vi "数字键盘.vi"(8 "错误输入":errorcluster caption="错误输入（无错误）", 11 "数值输入":string) -> (0 "错误输出":errorcluster, 3 "数值输出":string)   [LabVIEW 2014]
panel:
  in  "数字按钮":T1
  in  "放弃按钮":bool
  in  "删除":bool
  in  "清空":bool
  in  "确定按钮":bool
  in  "负号":bool
  in  "0":bool
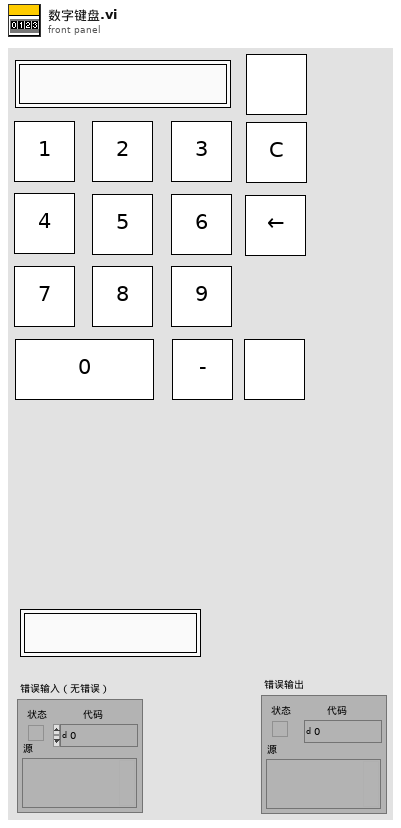
[diagram p1: front panel]
types:
  T1 = cluster{"1":bool, "2":bool, "3":bool, "4":bool, "5":bool, "6":bool, "7":bool, "8":bool, "9":bool}
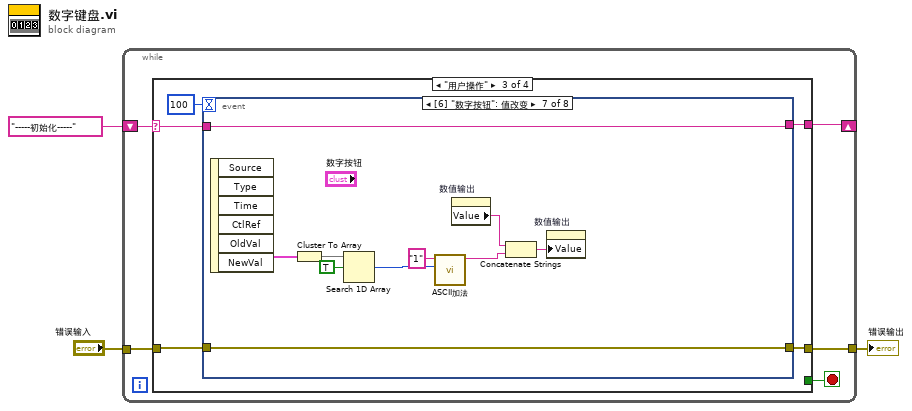
[diagram p0: block diagram]
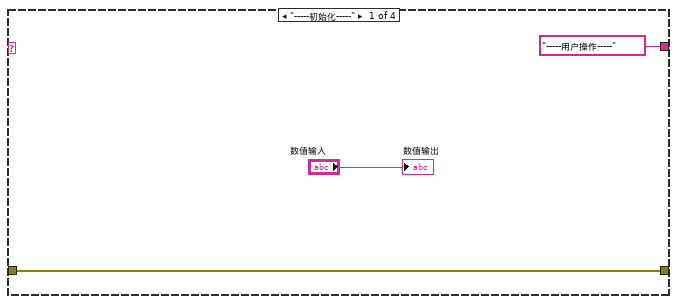
[diagram p2: hidden frame]
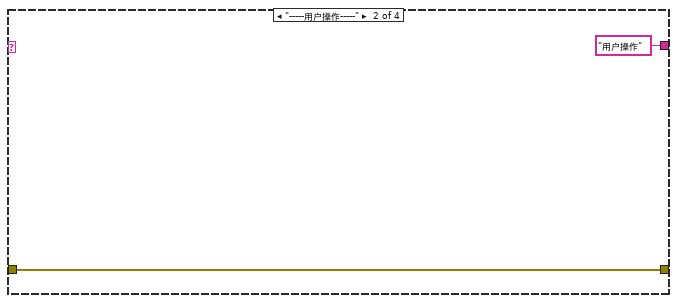
[diagram p3: hidden frame]
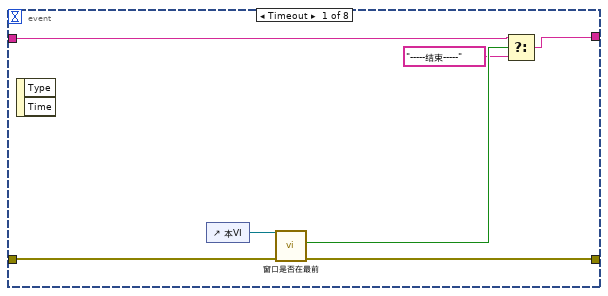
[diagram p4: hidden frame]
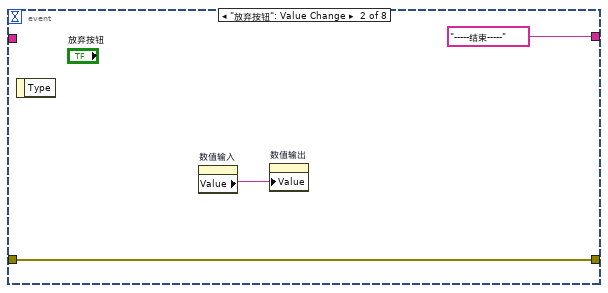
[diagram p5: hidden frame]
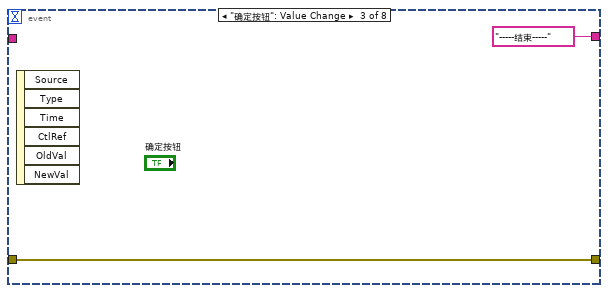
[diagram p6: hidden frame]
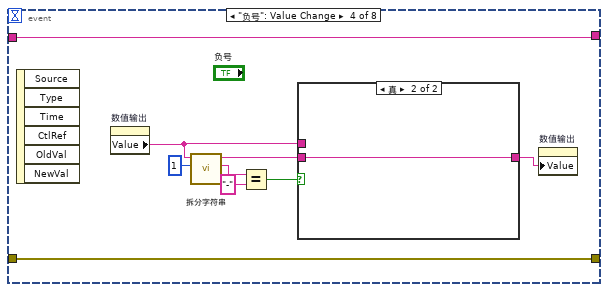
[diagram p7: hidden frame]
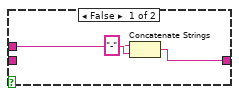
[diagram p8: hidden frame]
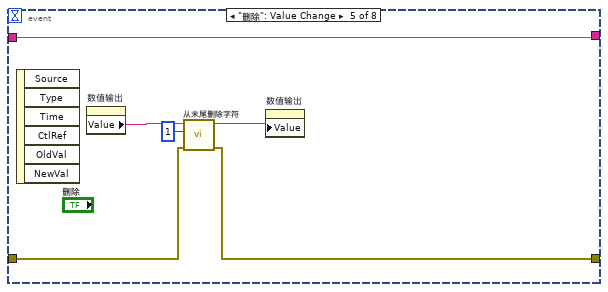
[diagram p9: hidden frame]
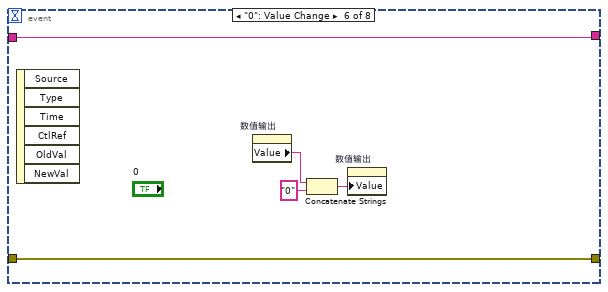
[diagram p10: hidden frame]
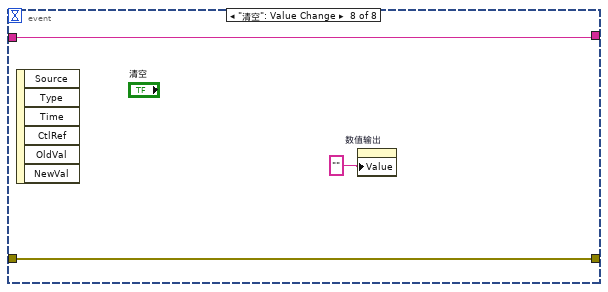
[diagram p11: hidden frame]
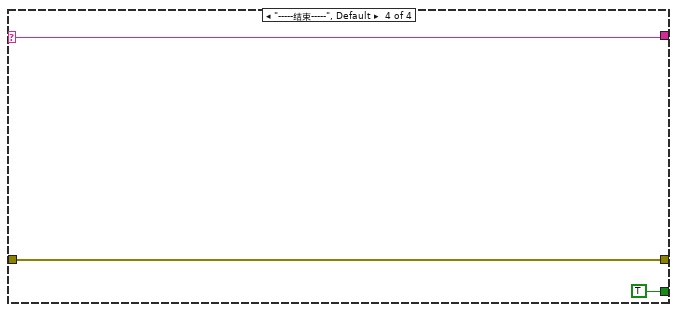
[diagram p12: hidden frame]
diagram:
  n1 = while {
    tunnel: [w8] -> w2
    tunnel: "错误输入" -> [w7]
    shift-right: [w4] -> _
    shift-left: "-----初始化-----" -> [w6]
    stop <- w5 stop-if-true
    n2 = case shown="\"用户操作\"" w6 {
      selector: w6 -> [_ _ w15 w68]
      tunnel: [w11 w12 w18 w70] -> w8
      tunnel: w7 -> [w11 w12 w17 w70]
      tunnel: [_ _ _ TRUE] -> w5
      tunnel: ["-----用户操作-----" "用户操作" w16 w68] -> w4
      frame "-----初始化-----" {
        "数值输出" <- "数值输入"
      }
      frame "-----用户操作-----" {
      }
      frame "用户操作" {
        n3 = event shown="[6] \"数字按钮\": 值改变" {
          selector: _ -> [_ _ _ _ _ _ _ _]
          dyn-events: _ -> [_ _ _ _ _ _ _ _]
          timeout: 100 -> [_ _ _ _ _ _ _ _]
          tunnel: [w24 w27 w30 w38 w45 w53 w64 w66] -> w18
          tunnel: w17 -> [w25 w27 w30 w38 w46 w53 w64 w66]
          tunnel: [w21 "-----结束-----" "-----结束-----" w39 w49 w54 w63 w67] -> w16
          tunnel: w15 -> [w22 _ _ w39 w49 w54 w63 w67]
          event Timeout {
            n4 = event-data() -> ()  [unwired: 1 in, 2 out]
            n5 = control-ref of="本VI"() -> (w19:refnum<vi>)
            n6 = call "窗口是否在最前.vi"("错误输入（无错误）"=w25, "引用"=w19) -> ("错误输出"=w24:errorcluster, "在最前？"=w23:bool)  [unwired: 7 in, 1 out]
            n7 = Select(t=w22, s=w23, f="-----结束-----") -> (s? t:f=w21:string)
          }
          event "放弃按钮": Value Change {
            n8 = event-data() -> ()  [unwired: 1 in, 1 out]
            n9 = property on="数值输入" class="Str"() -> ("Value"=w26:string)  [unwired: 2 in, 2 out]
            n10 = property on="数值输出" class="Str"("Value"=w26) -> ()  [unwired: 2 in, 2 out]
          }
          event "确定按钮": Value Change {
            n11 = event-data() -> ()  [unwired: 1 in, 6 out]
          }
          event "负号": Value Change {
            n12 = event-data() -> ()  [unwired: 1 in, 6 out]
            n13 = property on="数值输出" class="Str"() -> ("Value"=w31:string)  [unwired: 2 in, 2 out]
            n14 = call "拆分字符串.vi"("索引"=1, "字符串"=w31) -> ("拆分前"=w36:string, "剩余"=w32:string)  [unwired: 7 in, 1 out]
            n15 = Equal?(x=w36, y="-") -> (x = y?=w34:bool)
            n16 = case shown="真" w34 {
              tunnel: [w42 w43] -> w33
              tunnel: w32 -> [_ w43]
              tunnel: w31 -> [w41 _]
              frame False {
                n17 = Concatenate Strings("-" ("字符串"), w41) -> (w42:string)
              }
              frame True {
              }
            }
            n18 = property on="数值输出" class="Str"("Value"=w33) -> ()  [unwired: 2 in, 2 out]
          }
          event "删除": Value Change {
            n19 = event-data() -> ()  [unwired: 1 in, 6 out]
            n20 = property on="数值输出" class="Str"() -> ("Value"=w48:string)  [unwired: 2 in, 2 out]
            n21 = call "从末尾删除字符.vi"("error in (no error)"=w46, "删除位数"=1, "字符串输入"=w48) -> ("error out"=w45:errorcluster, "字符串输出"=w44:string)  [unwired: 7 in]
            n22 = property on="数值输出" class="Str"("Value"=w44) -> ()  [unwired: 2 in, 2 out]
          }
          event "0": Value Change {
            n23 = event-data() -> ()  [unwired: 1 in, 6 out]
            n24 = property on="数值输出" class="Str"() -> ("Value"=w51:string)  [unwired: 2 in, 2 out]
            n25 = Concatenate Strings(w51, "0" ("字符串")) -> (w50:string)
            n26 = property on="数值输出" class="Str"("Value"=w50) -> ()  [unwired: 2 in, 2 out]
          }
          event "数字按钮": Value Change {
            n27 = event-data() -> ("NewVal"=w62:T1)  [unwired: 1 in, 5 out]
            n28 = Cluster To Array(cluster=w62) -> (array=w61:bool[])
            n29 = Search 1D Array(1D array=w61, element=TRUE ("元素")) -> (index of element=w59:i32)  [unwired: 1 in]
            n30 = call-poly "ASCII加法.vi"("加数"=w59, "字符输入"="1") -> ("字符输出"=w57:string)  [unwired: 8 in, 1 out]
            n31 = property on="数值输出" class="Str"() -> ("Value"=w56:string)  [unwired: 2 in, 2 out]
            n32 = Concatenate Strings(w56, w57) -> (w55:string)
            n33 = property on="数值输出" class="Str"("Value"=w55) -> ()  [unwired: 2 in, 2 out]
          }
          event "清空": Value Change {
            n34 = event-data() -> ()  [unwired: 1 in, 6 out]
            n35 = property on="数值输出" class="Str"("Value"="" ("数值输出")) -> ()  [unwired: 2 in, 2 out]
          }
        }
      }
      frame "-----结束-----", Default {
      }
    }
  }
  "错误输出" <- w2
